vi "ETL Search Modules.vi"(7 "Limit":u32=10, 8 "error in (no error)":errorcluster, 9 "Module Type":string(combo), 10 "Site Name":string(combo), 11 "Base URL":string="https://staging-etl.app.cern.ch") -> (0 "error out":errorcluster, 3 "Search Result":T1)   [LabVIEW 2024, in "ETL API.lvlib"]
uses:
  ETL API.lvlib
  ETL API Search Result.ctl
  ETL Search Element.ctl
  <vilib>/addons/_JKI.lib/REST Client/classes/REST Client/REST Client.lvclass
panel:
  out "URL":string
  out "Response body":string
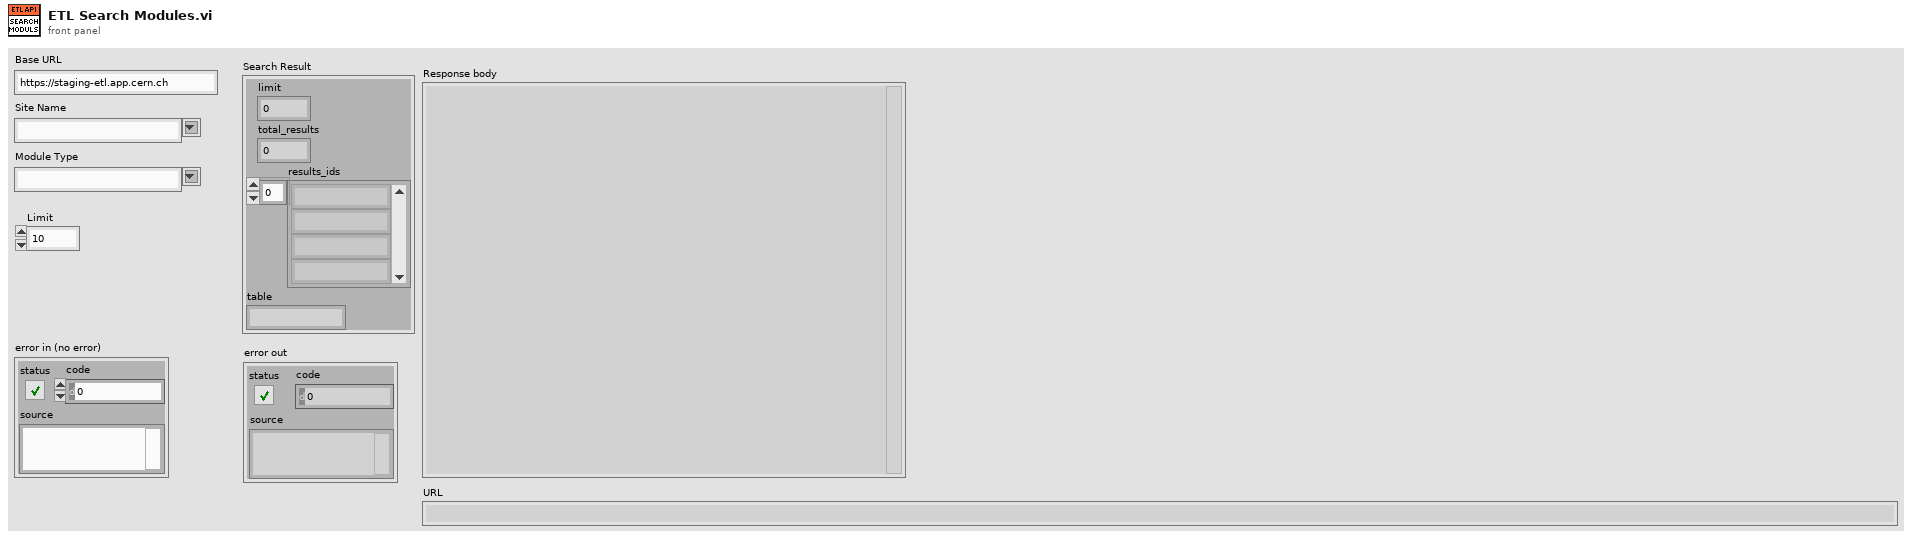
[diagram p1: front panel]
types:
  T1 = typedef "ETL API.lvlib/ETL API Search Result.ctl" = cluster{"limit":i32, "total_results":i32, "results_ids":string[], "table":string}
  T2 = typedef "ETL API.lvlib/ETL Search Element.ctl" = cluster{"Field":string, "Operator":string, "Value":string}
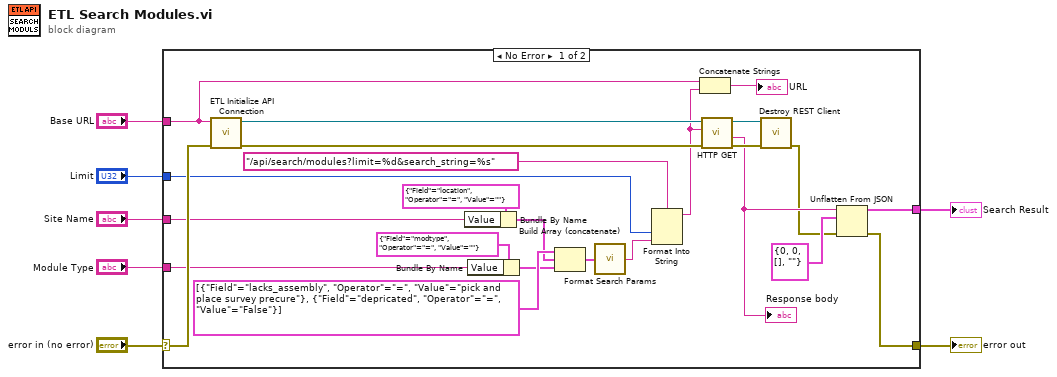
[diagram p0: block diagram]
diagram:
  n1 = case shown="No Error" "error in (no error)" {
    selector: "error in (no error)" -> [w29 w32]
    tunnel: "Base URL" -> [w14 _]
    tunnel: "Site Name" -> [w26 _]
    tunnel: [w15 w32] -> w4
    tunnel: "Module Type" -> [w24 _]
    tunnel: [w8 _] -> w2
    tunnel: "Limit" -> [w9 _]
    frame No Error {
      n2 = call "ETL Initialize API Connection.vi"("error in (no error)"=w29, "Base URL"=w14) -> ("error out"=w19:errorcluster, "REST Client out"=w28:refnum<class "REST Client.lvclass">)  [unwired: 8 in]
      n3 = Bundle By Name(cluster=T2 {"Field"="location", "Operator"="=", "Value"=""} ("ETL Search Element"), "Value"=w26) -> (w22:T2)
      n4 = Bundle By Name(cluster=T2 {"Field"="modtype", "Operator"="=", "Value"=""} ("ETL Search Element"), "Value"=w24) -> (w21:T2)
      n5 = Build Array (concatenate)(T2[] [{"Field"="lacks_assembly", "Operator"="=", "Value"="pick and place survey precure"}, {"Field"="depricated", "Operator"="=", "Value"="False"}], w22, w21) -> (w20:T2[])
      n6 = call "Format Search Params.vi"("Search Items"=w20) -> ("URL Param String"=w10:string)  [unwired: 3 in, 1 out]
      n7 = Format Into String(format string="/api/search/modules?limit=%d&search_string=%s" ("string"), w9, w10) -> (resulting string=w11:string)  [unwired: 2 in, 1 out]
      n8 = Concatenate Strings(w14, w11) -> (→"URL":string)
      n9 = call-dynamic "HTTP GET.vi"("error in (no error)"=w19, "Path"=w11, "REST Client in"=w28) -> ("error out"=w30:errorcluster, "Response body"=w18:string, "REST Client out"=w31:refnum<class "REST Client.lvclass">)  [unwired: 3 in, 3 out]
      "Response body" <- w18
      n10 = call-dynamic "Destroy REST Client.vi"("error in (no error)"=w30, "REST Client in"=w31) -> ("error out"=w16:errorcluster)  [unwired: 9 in]
      n11 = Unflatten From JSON(JSON string=w18, type and defaults=T1 {"limit"=0, "total_results"=0, "results_ids"=[], "table"=""} ("Search Result"), error in (no error)=w16) -> (value=w8:T1, error out=w15:errorcluster)  [unwired: 4 in]
    }
    frame Error {
    }
  }
  "error out" <- w4
  "Search Result" <- w2
